vi "getChannel.vi"(8 "error in (no error)":errorcluster, 9 "Channel":u16, 11 "Instrument.Amplifier in":refnum<class "Instrument.Amplifier.lvclass">) -> (0 "error out":errorcluster, 2 "channelProperties":variant, 3 "Instrument.Amplifier out":refnum<class "Instrument.Amplifier.lvclass">)   [LabVIEW 2019, in "Instrument.Amplifier.lvclass"]
uses:
  Instrument.Amplifier.lvclass
  Amplifier.Commands--Enum.ctl
  f9c57ccb-2530-4ad3-af3f-eaf4d6775a6f.vi
  f9c57ccb-2530-4ad3-af3f-eaf4d6775a6f.vi/a88c26e3-4d3b-485d-9d1e-7cdf6cefa23c.vi
  f9c57ccb-2530-4ad3-af3f-eaf4d6775a6f.vi/f6a8d593-a91c-4b3b-acb8-05b845705931.vi
  <vilib>/Utility/Data Type/Get Type Information.vi
  <vilib>/JDP Science/JSONtext/JSON text to Variant.vi
  <vilib>/JDP Science/JSONtext/LVClass Serializer/JSONtext LVClass Serializer.lvclass
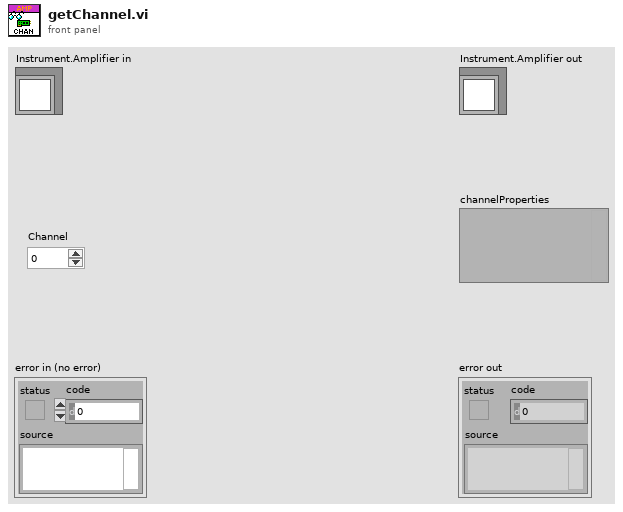
[diagram p1: front panel]
types:
  T1 = typedef "Instrument.Amplifier.lvclass/Amplifier.Commands--Enum.ctl" = enum16{"getChannel", "getAllChannels", "setChannel", "setAllChannels"}
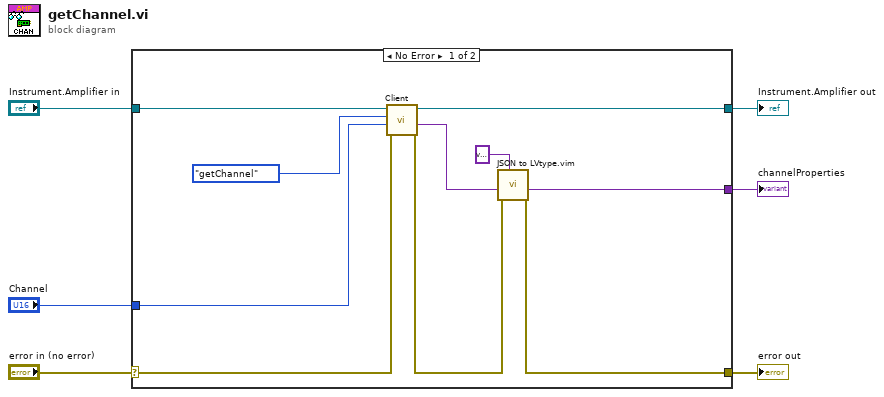
[diagram p0: block diagram]
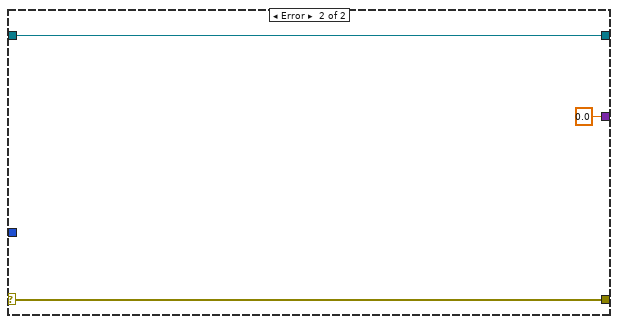
[diagram p2: hidden frame]
diagram:
  n1 = case shown="No Error" "error in (no error)" {
    selector: "error in (no error)" -> [w14 w19]
    tunnel: [w11 w19] -> w5
    tunnel: [w16 w18] -> w3
    tunnel: "Instrument.Amplifier in" -> [w7 w18]
    tunnel: [w10 0.0 ("Data out")] -> w2
    tunnel: "Channel" -> [w15 _]
    frame No Error {
      n2 = call-dynamic "Client.vi"("error in (no error)"=w14, "Data in"=w15, "Command in"=Amplifier.Commands--Enum."getChannel" ("Commands"), "Instrument in"=w7) -> ("error out"=w12:errorcluster, "Data out"=w13:variant, "Instrument out"=w16:refnum<class "Instrument.Amplifier.lvclass">)  [unwired: 4 in, 1 out]
      n3 = call "JSON to LVtype.vim"("type"=variant, "error in (no error)"=w12, "JSON Data in"=w13) -> ("error out"=w11:errorcluster, "Data out"=w10:variant)  [unwired: 7 in]
    }
    frame Error {
    }
  }
  "error out" <- w5
  "Instrument.Amplifier out" <- w3
  "channelProperties" <- w2
